vi "02-test.vi"() -> ()   [LabVIEW 2015]
panel:
  out "(hi.lo)":u32 format="%x"
  in  "hi":u8 format="%x"
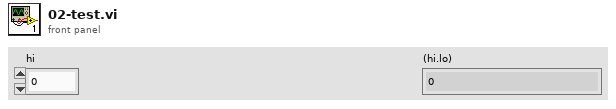
[diagram p1: front panel]
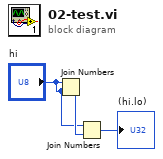
[diagram p0: block diagram]
diagram:
  n1 = Join Numbers(hi="hi", lo="hi") -> ((hi.lo)=w3:u16)
  n2 = Join Numbers(hi="hi", lo=w3) -> ((hi.lo)=→"(hi.lo)":u32)
